vi "TDMS Open.vi"(8 "error in (no error)":errorcluster, 11 "File Path Control":path=path "/home/lvuser/data") -> (0 "error out":errorcluster, 2 "TDMS file path string":path, 3 "tdms file out":refnum<k34>)   [LabVIEW 2015]
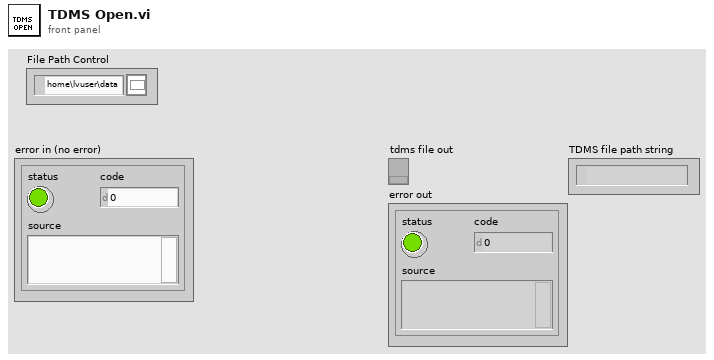
[diagram p1: front panel]
types:
  T1 = enum16{"open", "open or create", "create or replace", "create", "open (read-only)"}
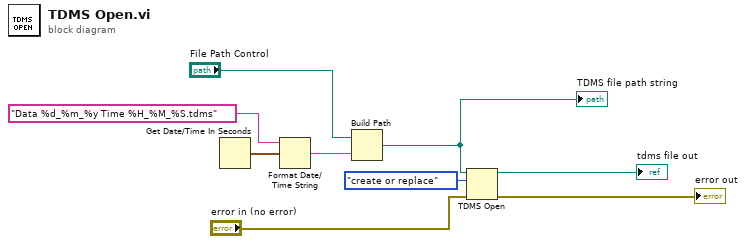
[diagram p0: block diagram]
diagram:
  n1 = Get Date/Time In Seconds() -> (seconds since 1Jan1904=w9:timestamp)
  n2 = Format Date/Time String(time format string (%c)="Data %d_%m_%y Time %H_%M_%S.tdms", seconds (now)=w9) -> (date/time string=w6:string)  [unwired: 1 in]
  n3 = Build Path(base path="File Path Control", name or relative path=w6) -> (appended path=w5:path)
  "TDMS file path string" <- w5
  n4 = TDMS Open(8:"error in (no error)", 10:T1."create or replace" ("operation (0:open)"), 11:w5) -> (0:→"error out":errorcluster, 3:→"tdms file out":refnum<k34>)  [unwired: 4 in]
